vi "YKMW100 DO Querry.vi"(0 "VISA session":refnum<visa-resource-name>="MW100", 2 "Semiphore":T1, 5 "Channel_Enum":T2=1 items=["4-20_OUT", "Pres_HI1", "Pres_HI2", "Pres_LOW", "Pres_PIN", "HEATER_TOP", "HEATER_BOT", "T_Shell", "FLOWMETER", "WATT_SENSE", "WH_TICK", "Tc_1", "Tc_2", "Tc_3", "Tc_4", "Tc_5", "Tc_6", "Tc_down", "T_Shell_2", "T_Shell_3", "T_Shell_4", "RTD_IN", "RTD_OUT", "RTD_AMB", "INTF_TEMPFLO", "INTF_READY", "INTF_START", "INTF_STOP", "DRM_LOW", "DRM_HIGH", "PWR_MAIN", "VLV_DUMP", "VLV_OUT", "VLV_IN", "WATT_HOURS", "FLOW(SAMPLE)", "GALLONS", "FLOW(GPM)"], 11 "error in (no error)":errorcluster) -> (4 "dup VISA session":refnum<visa-resource-name>="MW100", 6 "DO Val(T=Closed)":bool, 15 "error out":errorcluster)   [LabVIEW 2009]
doc: "This VI changes the operation mode.\nThe effective operation mode is Setting Mode and Measurement Mode.\n\nSee also: command \"DS\"."
uses:
  ChannelSettings.ctl
panel:
  out "Local?":bool
  out "Read Buffer":string
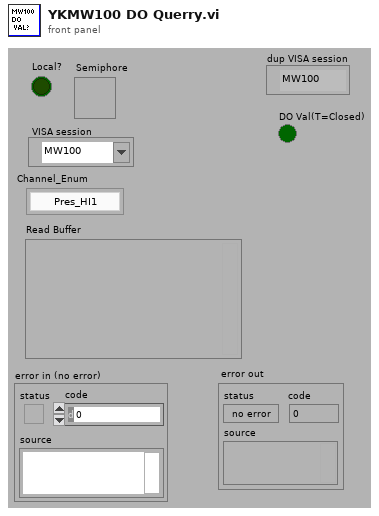
[diagram p1: front panel]
types:
  T1 = typedef "Semaphore RefNum" = refnum<k1>
  T2 = typedef "ChannelSettings.ctl" = u32
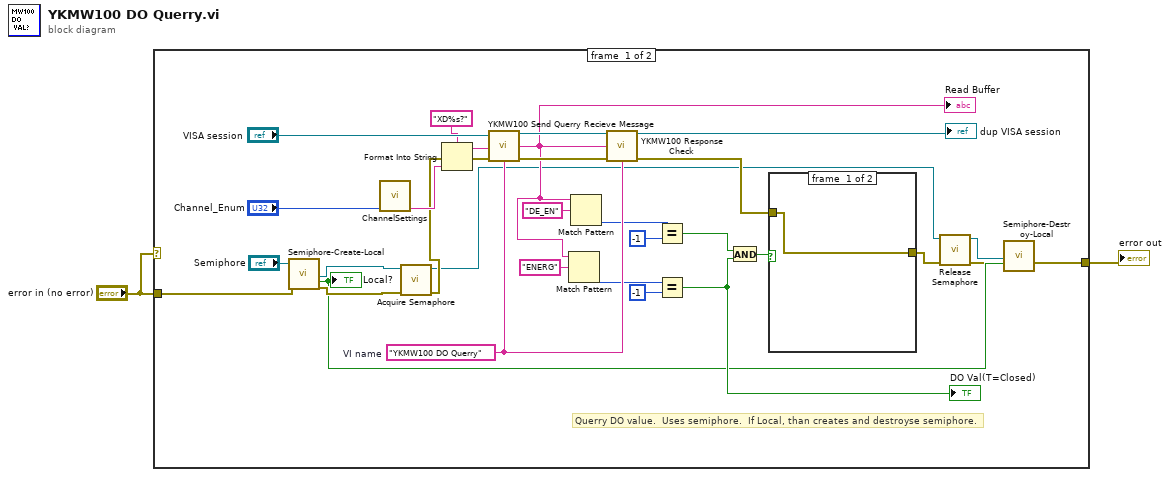
[diagram p0: block diagram]
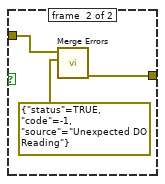
[diagram p2: hidden frame]
diagram:
  n1 = case shown="Error" "error in (no error)" {
    selector: "error in (no error)" -> [_ w38]
    tunnel: "error in (no error)" -> [w6 _]
    tunnel: [w3 w38] -> w2
    frame #0 {
      w26 = "YKMW100 DO Querry"  # VI name
      # "Querry DO value.  Uses semiphore.  If Local, than creates and destroyse semiphore."
      n2 = call "Semiphore-Create-Local.vi"("Semiphore"="Semiphore", "error in (no error)"=w6) -> ("semaphore"=w9:T1, "Local?"=w5:bool, "error out"=w8:errorcluster)  [unwired: 15 in]
      "Local?" <- w5
      n3 = call "ChannelSettings.vi"("Channel_Enum"="Channel_Enum") -> ("Channel String"=w25:string)  [unwired: 10 in]
      n4 = call <vilib>:"Acquire Semaphore.vi"("error in (no error)"=w8, "semaphore"=w9) -> ("error out"=w12:errorcluster, "semaphore out"=w10:T1)  [unwired: 3 in, 1 out]
      n5 = Format Into String(format string="XD%s?", error in=w12, w25) -> (resulting string=w30:string, error out=w32:errorcluster)  [unwired: 1 in]
      n6 = call "YKMW100 Send Querry Recieve Message.vi"("VISA session"="VISA session", "Send Message (\"\")"=w30, "error in (no error)"=w32, "Source (\"\")"=w26) -> ("dup VISA session"=w29:refnum<visa-resource-name>, "Read Buffer"=w22:string, "error out"=w28:errorcluster)  [unwired: 9 in]
      "Read Buffer" <- w22
      n7 = Match Pattern(string=w22, regular expression="ENERG") -> (offset past match=w18:i32)  [unwired: 1 in, 3 out]
      n8 = Match Pattern(string=w22, regular expression="DE_EN") -> (offset past match=w21:i32)  [unwired: 1 in, 3 out]
      n9 = call "YKMW100 Response Check.vi"("VISA session"=w29, "Message In (\"\")"=w22, "error in (no error)"=w28, "Source (\"\")"=w26) -> ("dup VISA session"=→"dup VISA session":refnum<visa-resource-name>, "error out"=w14:errorcluster)  [unwired: 7 in, 3 out]
      n10 = Equal?(x=w21, y=-1) -> (x = y?=w17:bool)
      n11 = Equal?(x=w18, y=-1) -> (x = y?=w16:bool)
      "DO Val(T=Closed)" <- w16
      n12 = And(x=w17, y=w16) -> (x .and. y?=w15:bool)
      n13 = case shown="False" w15 {
        tunnel: [w34 w37] -> w11
        tunnel: w14 -> [w34 w36]
        frame #0 {
        }
        frame #1 {
          n14 = call <vilib>:"Merge Errors.vi"("error in 2 (no error)"=errorcluster {"status"=TRUE, "code"=-1, "source"="Unexpected DO Reading"}, "error in 1 (no error)"=w36) -> ("error out"=w37:errorcluster)  [unwired: 5 in]
        }
      }
      n15 = call <vilib>:"Release Semaphore.vi"("error in (no error)"=w11, "semaphore"=w10) -> ("error out"=w3:errorcluster, "semaphore out"=w4:T1)  [unwired: 4 in]
      n16 = call "Semiphore-Destroy-Local.vi"("Semiphore"=w4, "Local?"=w5) -> ()  [unwired: 17 in, 1 out]
    }
    frame #1 {
    }
  }
  "error out" <- w2
